vi "Utility - Delete Files.vi"() -> ()   [LabVIEW 2015]
uses:
  <vilib>/nisyscfg/Filter Mode.ctl
  <vilib>/nisyscfg/Find Hardware.vi
  <vilib>/nisyscfg/Close (System).vi
  <vilib>/nisyscfg/nisyscfg.lvlib
  <resource>/objmgr/nisysapi.rc
  Globals/Global - Configuration Options.vi
panel:
  out "数组":string[](array[string])
  in  "多项":T1(array[cluster])
  in  "树形":string(tree)
  out "数值":i32
  out "大小":i32
  out "系统硬件数":i32
  out "名称":string[](array[string])
  out "插槽":i32[](array[numeric])
  out "插槽数":i32[](array[numeric])
  out "资源名称":string[](array[string])
  out "error out":errorcluster caption="错误输出"
  out "读数3":dbl
  in  "error in (no error) 2":errorcluster caption="错误输入（无错误）"
  out "读数1":dbl
  out "读数2":dbl
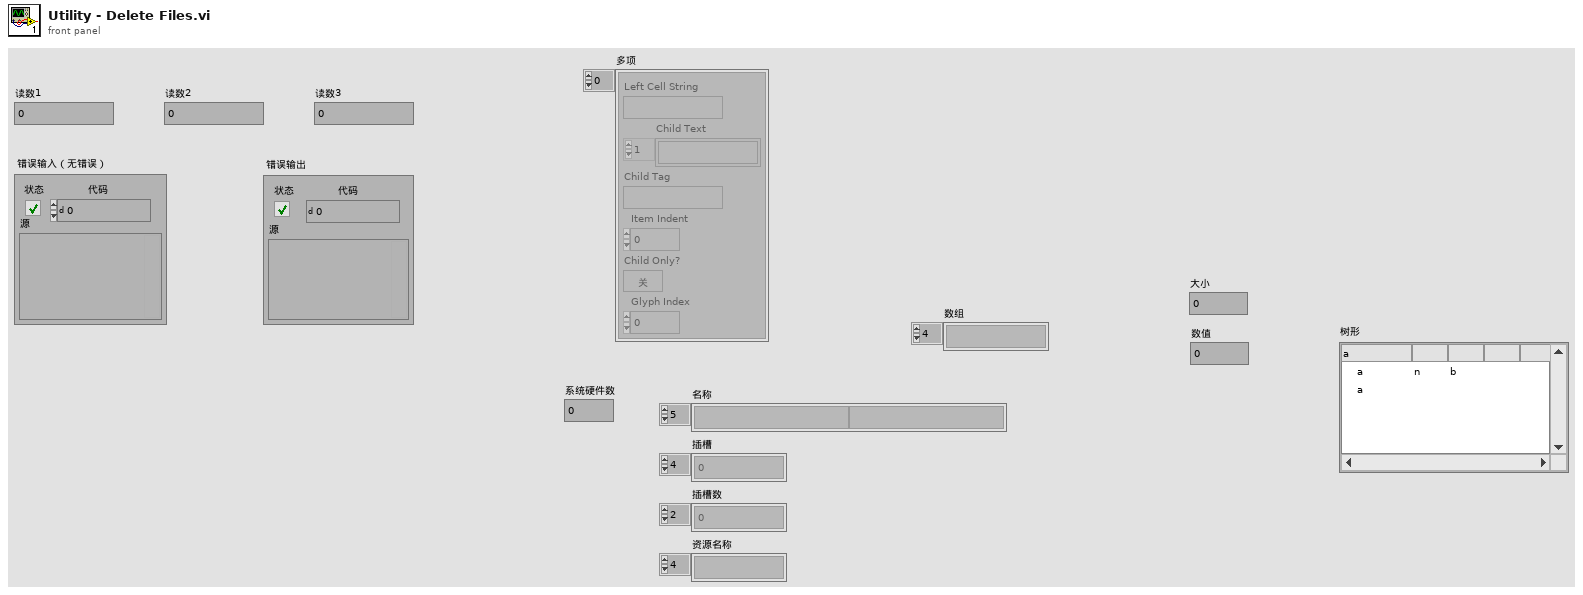
[diagram p1: front panel]
types:
  T1 = cluster{"Left Cell String":string, "Child Text":string[], "Child Tag":string, "Item Indent":i32, "Child Only?":bool, "Glyph Index":i32}[]
  T2 = typedef "nisyscfg.lvlib/Filter Mode.ctl" = i32
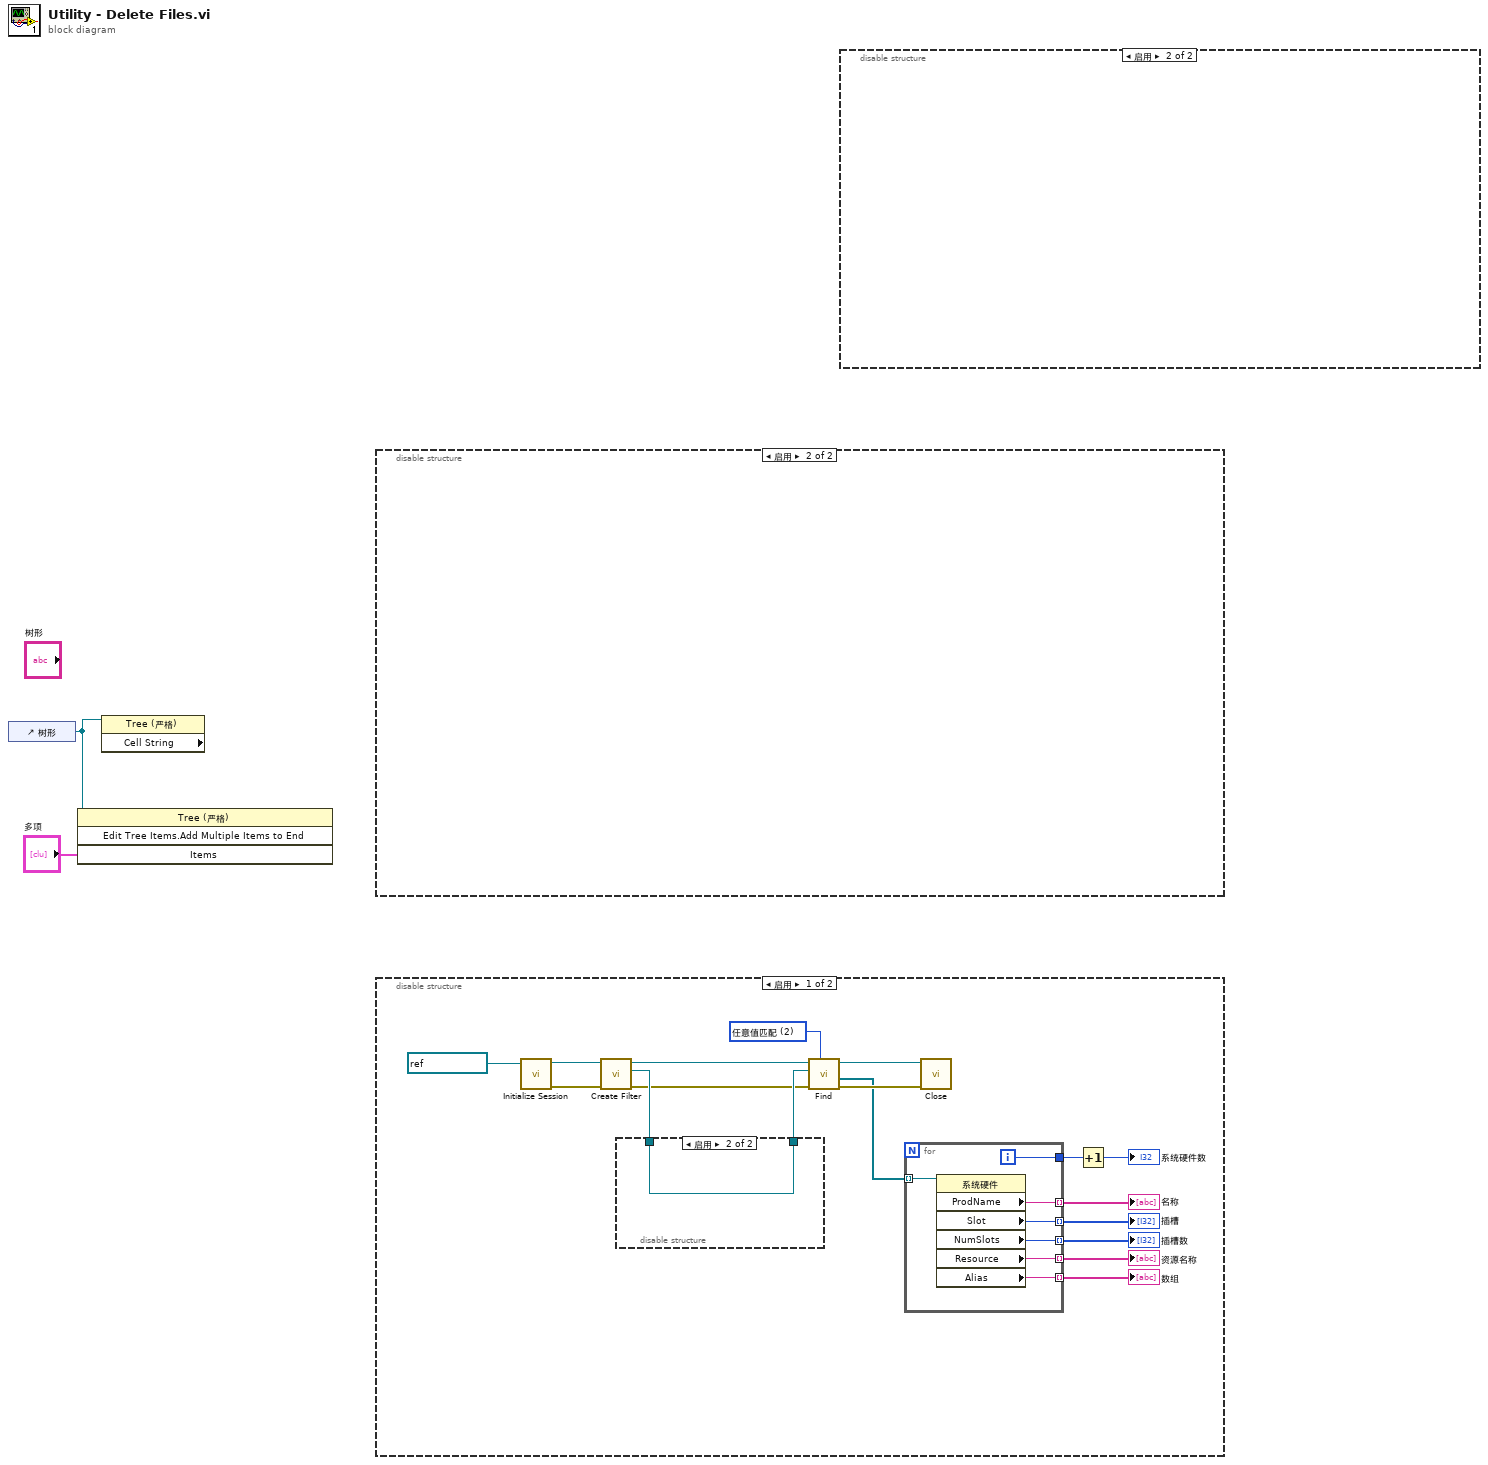
[diagram p0: block diagram]
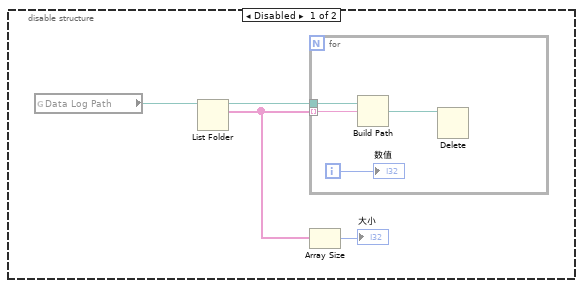
[diagram p2: hidden frame]
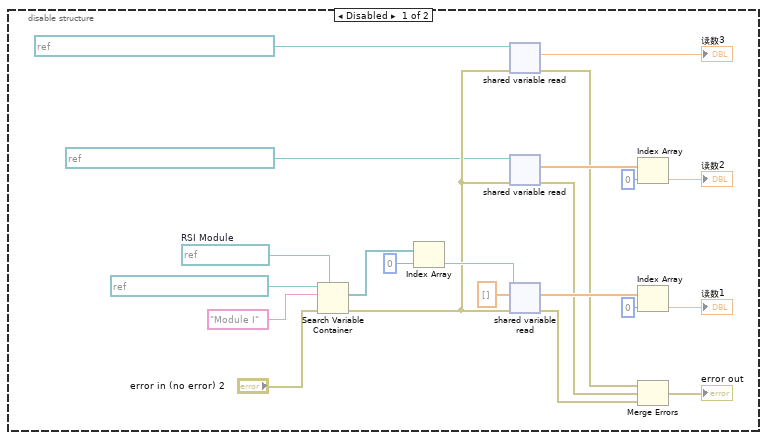
[diagram p3: hidden frame]
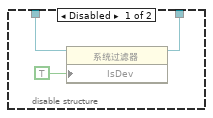
[diagram p4: hidden frame]
diagram:
  n1 = control-ref of="树形"() -> (w2:refnum<vi>)
  n2 = invoke class="Tree (严格)" method="Edit Tree Items.Add Multiple Items to End"(reference=w2, "Items"="多项") -> ()  [unwired: 2 in, 4 out]
  n3 = property class="Tree (严格)" props=["Cell String"](reference=w2) -> ()  [unwired: 1 in, 3 out]
  n4 = disable-structure shown="启用" {
    frame Disabled {
      w21 = refnum<k21> refnum  # RSI Module
      n5 = Search Variable Container(7:w21, 8:"error in (no error) 2", 10:"Module I" ("正则表达式"), 11:refnum<k21> "ni.var.io://169.254.4.42" ("容器引用句柄输入")) -> (0:w4:errorcluster, 2:w19:refnum<k21>[])  [unwired: 2 in, 1 out]
      n6 = Index Array(array=w19, index=0 ("索引")) -> (element=w17:refnum<k21>)
      n7 = shared-variable-read(refnum<k21> "ni.var.io://169.254.4.42/Module I/AI0" ("共享变量引用句柄输入"), w4) -> (w5:errorcluster, →"读数3":dbl)  [unwired: 1 out]
      n8 = shared-variable-read(refnum<k21> "ni.var.io://ni-crio9074/Module I" ("9234 constant"), w4) -> (w8:errorcluster, w24:dbl[])  [unwired: 1 out]
      n9 = shared-variable-read(w17, w4, dbl[] []) -> (w6:errorcluster, w14:dbl[])  [unwired: 1 out]
      n10 = Index Array(array=w24, index=0 ("索引")) -> (element=→"读数2":dbl)
      n11 = Index Array(array=w14, index=0 ("索引")) -> (element=→"读数1":dbl)
      n12 = Merge Errors(w5, w8, w6) -> (→"error out":errorcluster)
    }
    frame Enabled {
    }
  }
  n13 = disable-structure shown="启用" {
    frame Enabled {
      w37 = T2 2 items=["所有值匹配"=1, "任意值匹配"=2, "值不匹配"=3, "所有属性存在"=4] ("filter mode (all values match)")
      n14 = call <vilib>:"Initialize Session.vi"("Target (localhost)"=refnum<k21> "localhost" ("target (localhost)")) -> ("error out"=w42:errorcluster, "Session out"=w27:refnum<k21>)  [unwired: 9 in]
      n15 = call <vilib>:"Create Filter.vi"("error in (no error)"=w42, "Session in"=w27) -> ("error out"=w28:errorcluster, "Filter out"=w41:refnum<k20>, "Session out"=w29:refnum<k21>)  [unwired: 7 in]
      n16 = disable-structure shown="启用" {
        disable-tunnel: w41 -> [w45 w46]
        disable-tunnel: [w44 w46] -> w40
        frame Disabled {
          n17 = property class="系统过滤器"(reference=w45, "IsDev"=TRUE ("属于机箱")) -> (reference out=w44:refnum<k20>)  [unwired: 1 in, 1 out]
        }
        frame Enabled {
        }
      }
      n18 = call-poly <vilib>:"Find.vi"("Filter Mode (all values match)"=w37, "error in (no error)"=w28, "Filter in"=w40, "Session in"=w29) -> ("error out"=w39:errorcluster, "Resources out"=w36:refnum<k20>[], "Session out"=w38:refnum<k21>)  [unwired: 4 in, 1 out]
      n19 = for {
        tunnel: [w53] -> w33 mode=indexing
        tunnel: [w52] -> w32 mode=indexing
        tunnel: [w51] -> w31 mode=indexing
        tunnel: [w50] -> w30 mode=indexing
        tunnel: w36 -> [w49] mode=indexing
        tunnel: [w48] -> w35
        tunnel: [w47] -> w25 mode=indexing
        i -> [w48]
        n20 = property class="系统硬件"(reference=w49) -> ("ProdName"=w53:string, "Slot"=w52:i32, "NumSlots"=w51:i32, "Resource"=w50:string, "Alias"=w47:string)  [unwired: 1 in, 2 out]
      }
      "名称" <- w33
      "插槽" <- w32
      "插槽数" <- w31
      "资源名称" <- w30
      "数组" <- w25
      n21 = call-poly <vilib>:"Close.vi"("error in (no error)"=w39, "Session in"=w38) -> ()  [unwired: 9 in, 1 out]
      n22 = Increment(x=w35) -> (x+1=→"系统硬件数":i32)
    }
    frame Disabled {
    }
  }
  n23 = disable-structure shown="启用" {
    frame Disabled {
      n24 = global read "Global - Configuration Options.vi" "Data Log Path"() -> (w57:path)
      n25 = List Folder(path=w57) -> (path out=w56:path, filenames=w55:string[])  [unwired: 3 in, 2 out]
      n26 = for {
        tunnel: w55 -> [w60] mode=indexing
        tunnel: w56 -> [w61]
        i -> [w58]
        n27 = Build Path(base path=w61, name or relative path=w60) -> (appended path=w59:path)
        n28 = Delete(path (use dialog)=w59) -> ()  [unwired: 4 in, 3 out]
        "数值" <- w58
      }
      n29 = Array Size(array=w55) -> (size(s)=→"大小":i32)
    }
    frame Enabled {
    }
  }
